vi "CRYGet Current TS Steps.vi"(11 "Current Only?":bool) -> (0 "SelectStepNumber in Tree":i32, 1 "TS Name":string, 2 "EditStepName":string, 3 "Steps":T2[](array[typedef]) {"Repeat State Array"."Start" format="%#_5g"; "Y dB ref" format="%.1f"; "Y data" items=["dB", "Lin"]; "Start" format="%#_5g"}, 5 "TS Array":T1 {"Steps"."Repeat State Array"."Start" format="%#_5g"; "Steps"."Y dB ref" format="%.1f"; "Steps"."Y data" items=["dB", "Lin"]; "Steps"."Start" format="%#_5g"})   [LabVIEW 2013]
uses:
  CRYSystem/Typedef Control/CRYStep.ctl
  CRYSystem/Typedef Control/CRYTS.ctl
  CRYSystem/Calibration/SubVI/CRYCal Global.vi
  CRYProject Editor Global.vi
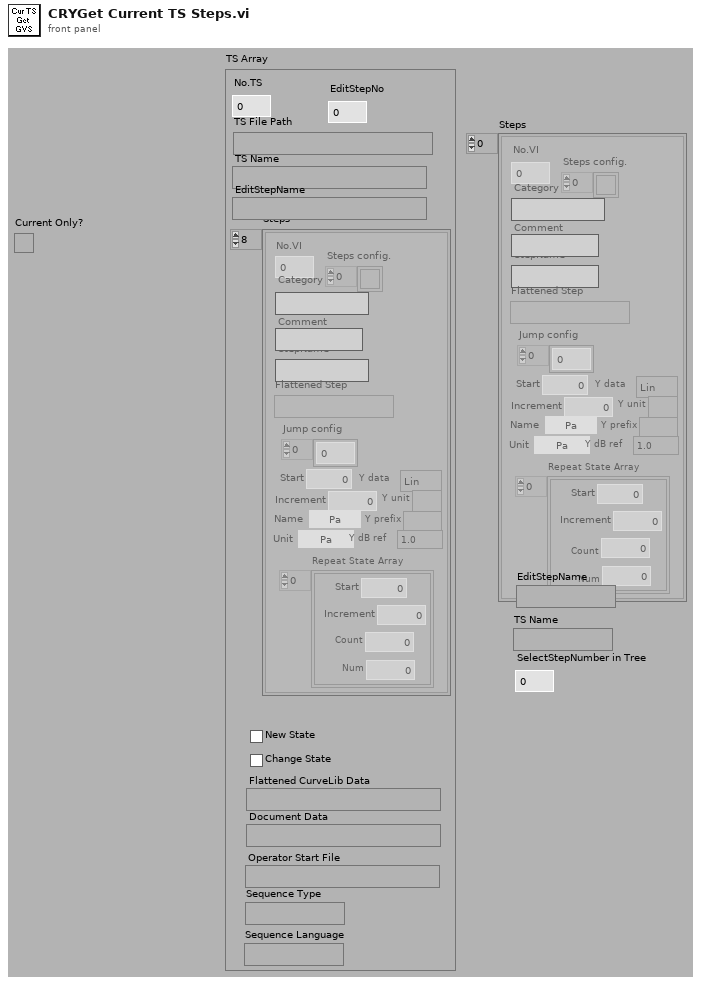
[diagram p1: front panel]
types:
  T1 = typedef "CRYTS.ctl" = cluster{"No.TS":u16, "TS File Path":path, "TS Name":string, "EditStepName":string, "Steps":T2[], "New State":bool, "Change State":bool, "Flattened CurveLib Data":string, "Document Data":string, "EditStepNo":u16, "Operator Start File":string, "Sequence Type":string, "Sequence Language":string}
  T2 = typedef "CRYStep.ctl" = cluster{"No.VI":i32, "Category":string, "StepName":string, "Seq setup flattened":string, "Comment":string, "Steps config.":bool[], "Jump config":i32[], "Start":dbl, "Increment":dbl, "Name":string, "Unit":string, "Y data":u16, "Y prefix":string, "Y dB ref":dbl, "Y unit":string, "Repeat State Array":cluster{"Start":dbl, "Increment":dbl, "Count":i32, "Num":i32}[]}
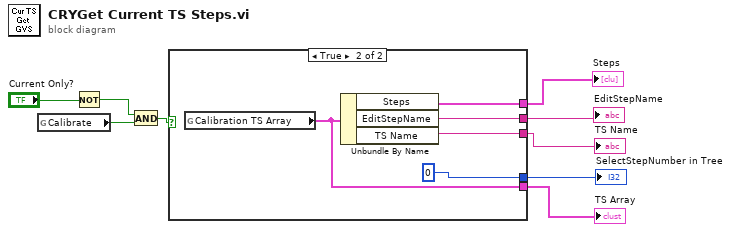
[diagram p0: block diagram]
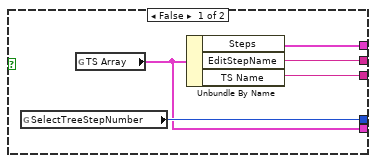
[diagram p2: hidden frame]
diagram:
  n1 = global read "CRYCal Global.vi" "Calibrate"() -> (w2:bool)
  n2 = Not(x="Current Only?") -> (.not. x?=w3:bool)
  n3 = And(x=w3, y=w2) -> (x .and. y?=w1:bool)
  n4 = case shown="True" w1 {
    tunnel: [w14 w19] -> w9
    tunnel: [w13 u16 0 ("SelectStepNumber")] -> w8
    tunnel: [w12 w17] -> w7
    tunnel: [w11 w16] -> w6
    tunnel: [w10 w15] -> w5
    frame False {
      n5 = global read "CRYProject Editor Global.vi" "SelectTreeStepNumber"() -> (w13:i32)
      n6 = global read "CRYProject Editor Global.vi" "TS Array"() -> (w10:T1)
      n7 = Unbundle By Name(w10) -> ("Steps"=w14:T2[], "EditStepName"=w12:string, "TS Name"=w11:string)
    }
    frame True {
      n8 = global read "CRYProject Editor Global.vi" "Calibration TS Array"() -> (w15:T1)
      n9 = Unbundle By Name(w15) -> ("Steps"=w19:T2[], "EditStepName"=w17:string, "TS Name"=w16:string)
    }
  }
  "Steps" <- w9
  "SelectStepNumber in Tree" <- w8
  "EditStepName" <- w7
  "TS Name" <- w6
  "TS Array" <- w5
